vi "labo01.02.vi"() -> ()   [LabVIEW 2020]
panel:
  out "slowo 8":string
  out "slowo 7":string
  out "slowo 6":string
  out "slowo 5":string
  out "slowo 4":string
  out "slowo 3":string
  out "slowo 2":string
  out "slowo":string
  in  "jaksięczłowiekśpieszy,tosiędiabełcieszy":string
  out "Poprawione zdanie:":string
  in  "Napisz zdanie:":string
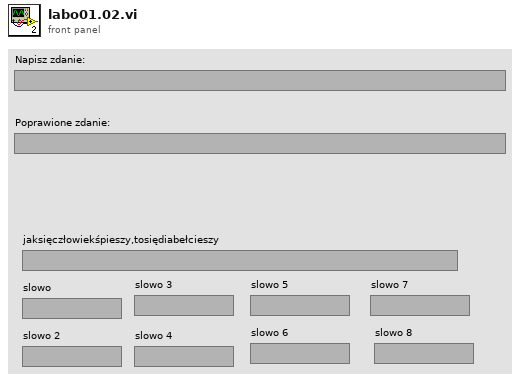
[diagram p1: front panel]
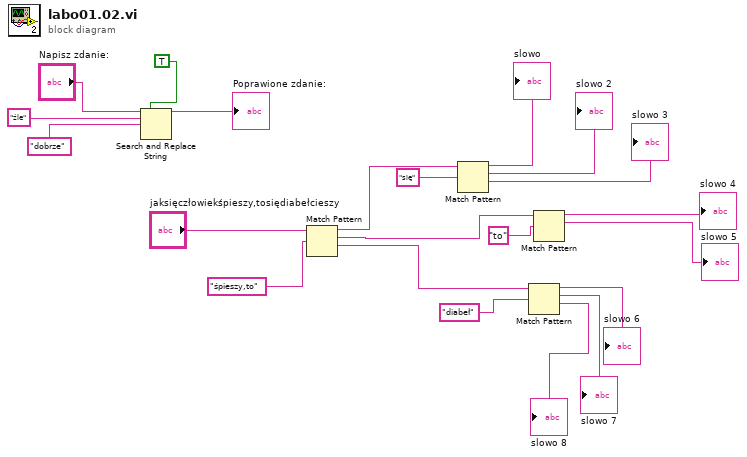
[diagram p0: block diagram]
diagram:
  n1 = Search and Replace String(replace all?=TRUE, input string="Napisz zdanie:", search string="źle", replace string="dobrze") -> (result string=→"Poprawione zdanie:":string)  [unwired: 4 in, 3 out]
  n2 = Match Pattern(string="jaksięczłowiekśpieszy,tosiędiabełcieszy", regular expression="śpieszy,to") -> (before substring=w14:string, match substring=w10:string, after substring=w11:string)  [unwired: 1 in, 1 out]
  n3 = Match Pattern(string=w14, regular expression="się") -> (before substring=→"slowo":string, match substring=→"slowo 2":string, after substring=→"slowo 3":string)  [unwired: 1 in, 1 out]
  n4 = Match Pattern(string=w11, regular expression="diabeł") -> (before substring=→"slowo 6":string, match substring=→"slowo 7":string, after substring=→"slowo 8":string)  [unwired: 1 in, 1 out]
  n5 = Match Pattern(string=w10, regular expression="to") -> (before substring=→"slowo 4":string, match substring=→"slowo 5":string)  [unwired: 1 in, 2 out]
